vi "RSZVB Get Port Power Generator Offset.vi"(7 "Generator Number (1)":i32=1, 8 "error in (no error)":errorcluster {"code" format="%.0x"}, 9 "Port Number (1)":i32=1, 10 "Channel (1)":i32=1, 11 "VISA session":refnum<visa-resource-name>) -> (0 "error out":errorcluster {"code" format="%.0x"}, 1 "Offset Parameter":i32, 2 "Port Power Offset":dbl format="%^.3e", 3 "dup VISA session":refnum<visa-resource-name>)   [LabVIEW 2011]
doc: "This VI queries the power of an external generator or its power offset relative to the channel power. \n\nNote(s):\n\n(1) This VI is available only on R&S ZVA instrument.\n\nRemote-control command(s):\nSOURce<Ch>:POWer<Pt>:GENerator<Gen>:OFFSet?"
uses:
  _utility/RSZVB Global Data.vi
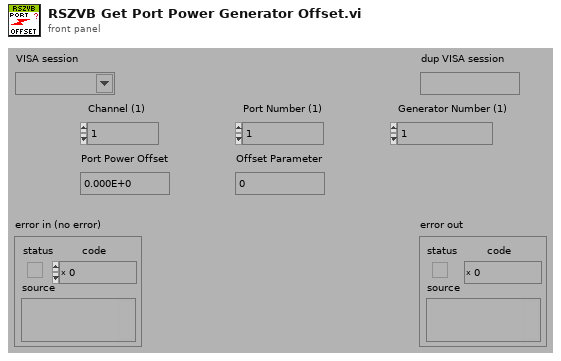
[diagram p1: front panel]
types:
  T1 = cluster{"Error Checking (T: On)":bool, "Installed Options":string[], "Data Valid?":bool, "Ports":i32, "Model":string[], "Option Checking (T: On)":bool}[]
  T2 = cluster{"Error Checking (T: On)":bool, "Installed Options":string[], "Data Valid?":bool, "Ports":i32, "Model":string[], "Option Checking (T: On)":bool}
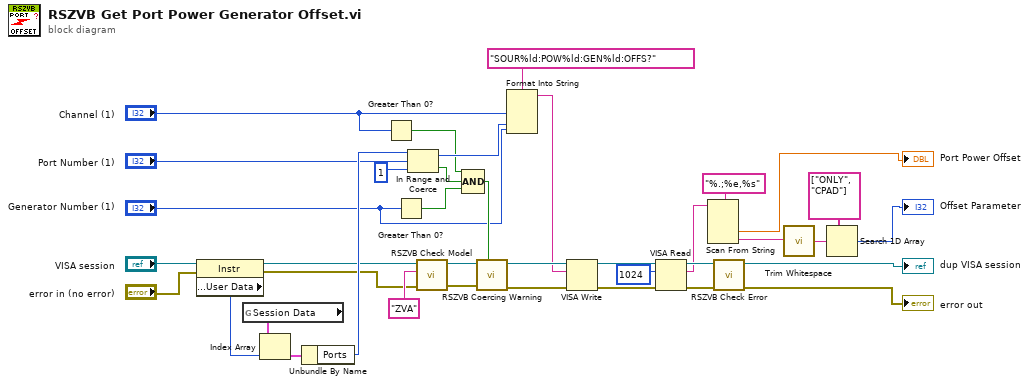
[diagram p0: block diagram]
diagram:
  n1 = property class="Instr"(reference="VISA session", error in="error in (no error)") -> (reference out=w2:refnum<visa-resource-name>, error out=w1:errorcluster, "General Settings:User Data"=w25:u32)
  n2 = global read "RSZVB Global Data.vi" "Session Data"() -> (w26:T1)
  n3 = Index Array(array=w26, index=w25) -> (element=w27:T2)
  n4 = Unbundle By Name(w27) -> ("Ports"=w23:i32)
  n5 = Greater Than 0?(x="Channel (1)") -> (x > 0?=w21:bool)
  n6 = Greater Than 0?(x="Generator Number (1)") -> (x > 0?=w7:bool)
  n7 = In Range and Coerce(upper limit=w23, x="Port Number (1)", lower limit=1) -> (coerced(x)=w22:i32, In Range?=w20:bool)
  n8 = call "RSZVB Check Model.vi"("error in (no error)"=w1, "Model"="ZVA" ("Options"), "VISA session"=w2) -> ("error out"=w3:errorcluster, "dup VISA session"=w4:refnum<visa-resource-name>)  [unwired: 7 in]
  n9 = Compound Arithmetic op=AND(w21, w20, w7) -> (w19:bool)
  n10 = call "RSZVB Coercing Warning.vi"("In Range?"=w19, "error in (no error)"=w3, "VISA session"=w4) -> ("error out"=w30:errorcluster, "dup VISA session"=w31:refnum<visa-resource-name>)  [unwired: 7 in]
  n11 = Format Into String(format string="SOUR%ld:POW%ld:GEN%ld:OFFS?", "Channel (1)", w22, "Generator Number (1)") -> (resulting string=w28:string)  [unwired: 2 in, 1 out]
  n12 = VISA Write(VISA resource name=w31, write buffer=w28, error in (no error)=w30) -> (VISA resource name out=w32:refnum<visa-resource-name>, error out=w33:errorcluster)  [unwired: 1 out]
  n13 = VISA Read(VISA resource name=w32, byte count=u32 1024 ("byte count (0)"), error in (no error)=w33) -> (VISA resource name out=w37:refnum<visa-resource-name>, read buffer=w34:string, error out=w36:errorcluster)  [unwired: 1 out]
  n14 = Scan From String(format string="%.;%e,%s", input string=w34) -> (output 1=→"Port Power Offset":dbl, output 2=w16:string)  [unwired: 4 in, 3 out]
  n15 = call "RSZVB Check Error.vi"("error in (no error)"=w36, "VISA session"=w37) -> ("error out"=→"error out":errorcluster, "dup VISA session"=→"dup VISA session":refnum<visa-resource-name>)  [unwired: 8 in]
  n16 = call <vilib>:"Trim Whitespace.vi"("string"=w16) -> ("trimmed string"=w17:string)  [unwired: 1 in]
  n17 = Search 1D Array(1D array=string[] ["ONLY", "CPAD"] ("array 2"), element=w17) -> (index of element=→"Offset Parameter":i32)  [unwired: 1 in]
